vi "dfd_FIR Spectral Factorization.vi"(8 "error in (no error)":errorcluster, 11 "H(n)":dbl[](array[numeric])) -> (0 "error out":errorcluster, 1 "H(n) 2":dbl[](array[numeric]), 2 "H(n) 1":dbl[](array[numeric]))   [LabVIEW 2017, in "NI_DigFilter_FilterBank.lvlib"]
doc: "Spectrally factorizes the <B>filter in</B> into two filters by specified method."
uses:
  <vilib>/addons/Digital Filter Design/NI_DigFilter_FilterBank.lvlib
  <vilib>/Analysis/2dsp.llb/1D Auto Correlation (DBL).vi
  <vilib>/addons/Digital Filter Design/_Misc.llb/dfd_Error Cluster From Error Code (Array).vi
  <vilib>/addons/Digital Filter Design/NI_DigFilter_Design.lvlib
  <vilib>/addons/Digital Filter Design/NI_DigFilterLicensed.lvlib
  <vilib>/Analysis/NI_AALPro.lvlib
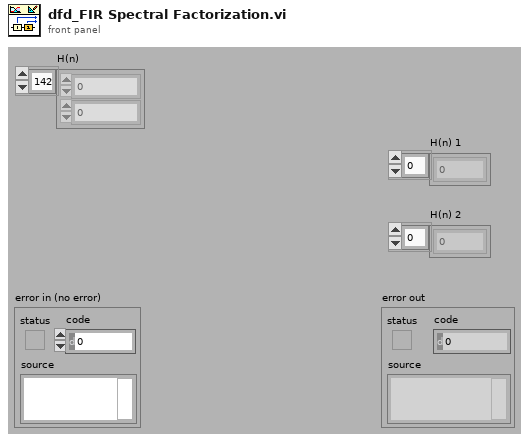
[diagram p1: front panel]
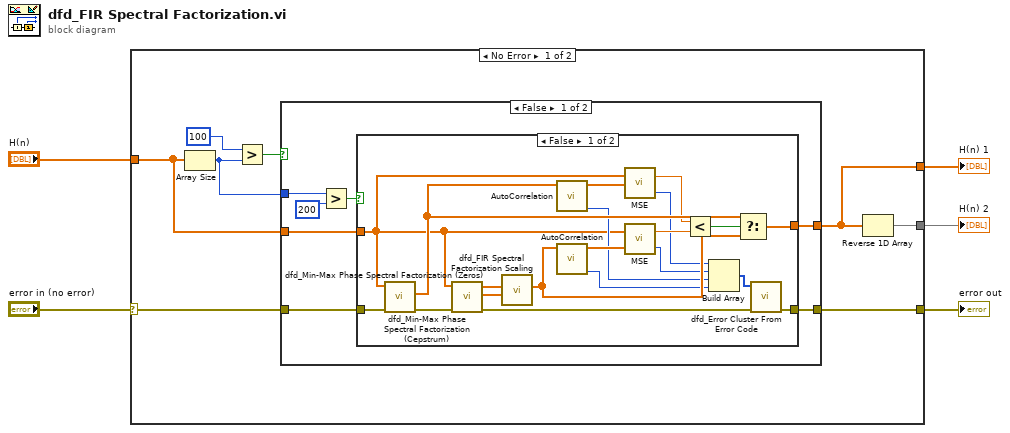
[diagram p0: block diagram]
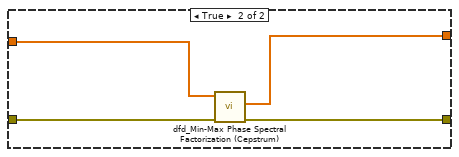
[diagram p2: hidden frame]
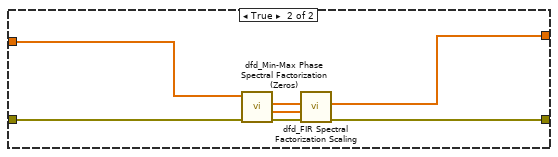
[diagram p3: hidden frame]
diagram:
  n1 = case shown="No Error" "error in (no error)" {
    selector: "error in (no error)" -> [w11 w51]
    tunnel: [w10 w51] -> w4
    tunnel: "H(n)" -> [w12 _]
    tunnel: [w13 _] -> w1
    tunnel: [w9 _] -> w2
    frame No Error {
      n2 = Array Size(array=w12) -> (size(s)=w6:i32)
      n3 = Greater?(x=100, y=w6) -> (0:w7:bool)
      n4 = case shown="False" w7 {
        tunnel: w12 -> [w20 w48]
        tunnel: [w19 w45] -> w13
        tunnel: w6 -> [w18 _]
        tunnel: w11 -> [w15 w49]
        tunnel: [w14 w50] -> w10
        frame False {
          n5 = Greater?(x=w18, y=200) -> (0:w16:bool)
          n6 = case shown="False" w16 {
            tunnel: w20 -> [w21 w44]
            tunnel: [w38 w43] -> w19
            tunnel: w15 -> [w37 w42]
            tunnel: [w33 w41] -> w14
            frame False {
              n7 = call <vilib>:"dfd_Min-Max Phase Spectral Factorization (Cepstrum).vi"("error in (no error)"=w37, "numerator"=w21) -> ("error out"=w36:errorcluster, "minimum phase"=w39:dbl[])  [unwired: 7 in, 1 out]
              n8 = call <vilib>:"dfd_Min-Max Phase Spectral Factorization (Zeros).vi"("error in (no error)"=w36, "numerator"=w21) -> ("error out"=w34:errorcluster, "maximum phase"=w27:dbl[], "minimum phase"=w28:dbl[])  [unwired: 7 in]
              n9 = call <vilib>:"dfd_FIR Spectral Factorization Scaling.vi"("maximum phase in"=w27, "minimum phase in"=w28) -> ("minimum phase"=w26:dbl[])  [unwired: 8 in, 1 out]
              n10 = call-poly <vilib>:"AutoCorrelation.vi"("X"=w39) -> ("error"=w23:i32, "Rxx"=w32:dbl[])  [unwired: 9 in]
              n11 = call-poly <vilib>:"AutoCorrelation.vi"("X"=w26) -> ("error"=w22:i32, "Rxx"=w30:dbl[])  [unwired: 9 in]
              n12 = call <vilib>:"MSE.vi"("X Values"=w32, "Y Values"=w21) -> ("error"=w25:i32, "mse"=w31:dbl)
              n13 = call <vilib>:"MSE.vi"("X Values"=w30, "Y Values"=w21) -> ("error"=w24:i32, "mse"=w29:dbl)
              n14 = Less?(x=w31, y=w29) -> (x < y?=w40:bool)
              n15 = Build Array(w25, w24, w23, w22) -> (w35:i32[])
              n16 = Select(t=w39, s=w40, f=w26) -> (s? t:f=w38:dbl[])
              n17 = call-poly <vilib>:"dfd_Error Cluster From Error Code.vi"("error in (no error)"=w34, "error code (0)"=w35) -> ("error out"=w33:errorcluster)  [unwired: 9 in]
            }
            frame True {
              n18 = call <vilib>:"dfd_Min-Max Phase Spectral Factorization (Cepstrum).vi"("error in (no error)"=w42, "numerator"=w44) -> ("error out"=w41:errorcluster, "minimum phase"=w43:dbl[])  [unwired: 7 in, 1 out]
            }
          }
        }
        frame True {
          n19 = call <vilib>:"dfd_Min-Max Phase Spectral Factorization (Zeros).vi"("error in (no error)"=w49, "numerator"=w48) -> ("error out"=w50:errorcluster, "maximum phase"=w46:dbl[], "minimum phase"=w47:dbl[])  [unwired: 7 in]
          n20 = call <vilib>:"dfd_FIR Spectral Factorization Scaling.vi"("maximum phase in"=w46, "minimum phase in"=w47) -> ("minimum phase"=w45:dbl[])  [unwired: 8 in, 1 out]
        }
      }
      n21 = Reverse 1D Array(array=w13) -> (reversed array=w9:dbl[])
    }
    frame Error {
    }
  }
  "error out" <- w4
  "H(n) 1" <- w1
  "H(n) 2" <- w2
